vi "WaveFilter.vi"(8 "错误输入（无错误）":errorcluster, 10 "FilterCoefficient":i32, 11 "Wave In":dbl) -> (0 "错误输出":errorcluster, 3 "Wave Out":dbl)   [LabVIEW 2020]
uses:
  DLL/WaveFilter/WaveFilter.dll
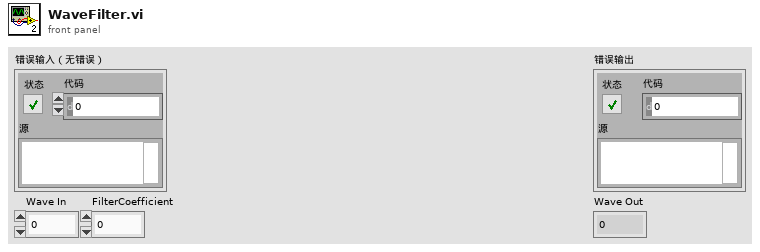
[diagram p1: front panel]
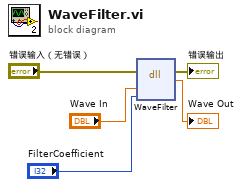
[diagram p0: block diagram]
diagram:
  n1 = dll-call lib="PTH2kabs CUsersFengDesktopC-EPS020芯轴分总成磨合台SourcesDLL\nWaveFilterWaveFilter.dll" fn="WaveFilter"(error in="错误输入（无错误）", "Wave In"="Wave In", "FilterCoefficient"="FilterCoefficient") -> (error out=→"错误输出":errorcluster, "返回类型"=→"Wave Out":dbl)  [unwired: 4 in, 1 out]
